vi "FRCts20_Backend_TeamRoot_GET.vi"(6 "Message Attributes":T4, 8 "error in (no error)":errorcluster, 10 "Data":string, 11 "Engine_Refnums":T1) -> (0 "error out":errorcluster)   [LabVIEW 2014, in "FRCts20_Backend_Engine.lvlib"]
doc: "Retrieves all team information, called by the Team Root API. No inputs expected"
uses:
  FRCts20_Backend_Engine.lvlib
  Dependencies/Keyed Array/KeyedArray.ctl
  FRCts20_Backend_EngineRefnums.ctl
  INI_Accessor/FRCts20_Backend_INI Controller.lvclass
  Dependencies/AMC/_SubVIs/TypeDefs/Message Queue.ctl
  Dependencies/AMC/_SubVIs/TypeDefs/Message.ctl
  <vilib>/addons/database/Connection.llb/Conn ObjectReference.ctl
  FRCts20_Backend_FGVOperation.ctl
  Dependencies/Keyed Array/Tools_KeyedArray.lvlib
  Dependencies/AMC/AMC.lvlib
  <vilib>/addons/database/NI_Database_API.lvlib
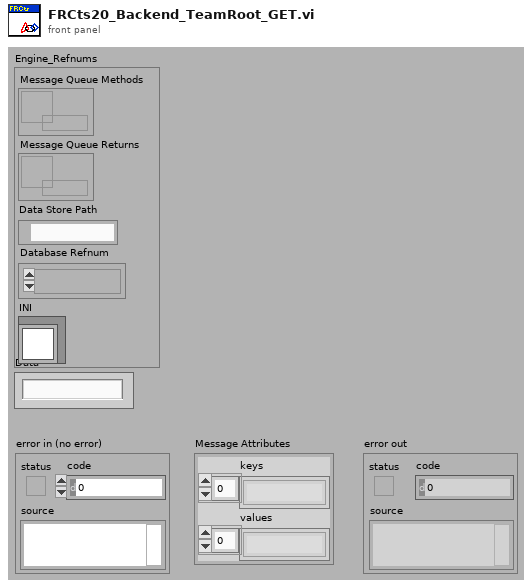
[diagram p1: front panel]
types:
  T1 = typedef "FRCts20_Backend_Engine.lvlib/FRCts20_Backend_EngineRefnums.ctl" = cluster{"Message Queue Methods":T2, "Message Queue Returns":T2, "Data Store Path":path, "Database Refnum":T3, "INI":refnum<class "FRCts20_Backend_INI Controller.lvclass">}
  T2 = typedef "AMC.lvlib/Message Queue.ctl" = refnum<queue>
  T3 = typedef "NI_Database_API.lvlib/Conn ObjectReference.ctl" = refnum<k1>
  T4 = typedef "Tools_KeyedArray.lvlib/KeyedArray.ctl" = cluster{"keys":string[], "values":string[]}
  T5 = typedef "FRCts20_Backend_Engine.lvlib/FRCts20_Backend_FGVOperation.ctl" = enum16{"Initialize", "EnqueueMessage", "EnqueueDataReturn", "FlushMessage", "FlushDataReturn"}
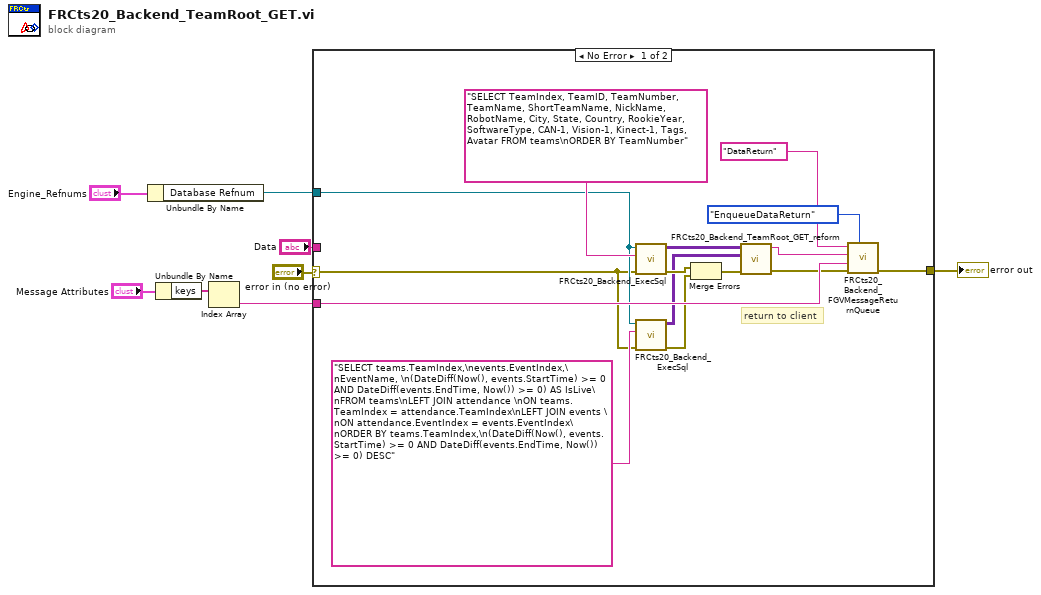
[diagram p0: block diagram]
diagram:
  n1 = Unbundle By Name("Engine_Refnums") -> ("Database Refnum"=w1:T3)
  n2 = Unbundle By Name("Message Attributes") -> ("keys"=w4:string[])
  n3 = Index Array(array=w4) -> (element=w3:string)  [unwired: 1 in]
  n4 = case shown="No Error" "error in (no error)" {
    selector: "error in (no error)" -> [w9 w24]
    tunnel: [w23 w24] -> w7
    tunnel: w1 -> [w13 _]
    tunnel: "Data" -> [_ _]
    tunnel: w3 -> [w22 _]
    frame No Error {
      # "return to client"
      n5 = call "FRCts20_Backend_ExecSql.vi"("error in (no error)"=w9, "format string"="SELECT TeamIndex, TeamID, TeamNumber, TeamName, ShortTeamName, NickName, RobotName, City, State, Country, RookieYear, SoftwareType, CAN-1, Vision-1, Kinect-1, Tags, Avatar FROM teams\nORDER BY TeamNumber", "Refnum in"=w13) -> ("error out"=w14:errorcluster, "recordset data"=w17:variant[][])  [unwired: 6 in, 1 out]
      n6 = call "FRCts20_Backend_ExecSql.vi"("error in (no error)"=w9, "format string"="SELECT teams.TeamIndex,\nevents.EventIndex,\nEventName, \n(DateDiff(Now(), events.StartTime) >= 0 AND DateDiff(events.EndTime, Now()) >= 0) AS IsLive\nFROM teams\nLEFT JOIN attendance \nON teams.TeamIndex = attendance.TeamIndex\nLEFT JOIN events \nON attendance.EventIndex = events.EventIndex\nORDER BY teams.TeamIndex,\n(DateDiff(Now(), events.StartTime) >= 0 AND DateDiff(events.EndTime, Now()) >= 0) DESC", "Refnum in"=w13) -> ("error out"=w11:errorcluster, "recordset data"=w10:variant[][])  [unwired: 6 in, 1 out]
      n7 = Merge Errors(w14, w11) -> (w15:errorcluster)
      n8 = call "FRCts20_Backend_TeamRoot_GET_reform.vi"("error in (no error)"=w15, "eventdata"=w10, "recordset data"=w17) -> ("error out"=w18:errorcluster, "data string"=w19:string)  [unwired: 7 in]
      n9 = call "FRCts20_Backend_FGVMessageReturnQueue.vi"("Operation"=FRCts20_Backend_FGVOperation."EnqueueDataReturn", "error in (no error)"=w18, "Key"=w22, "Message Value"=w19, "Message Name"="DataReturn") -> ("error out"=w23:errorcluster)  [unwired: 5 in, 1 out]
    }
    frame Error {
    }
  }
  "error out" <- w7
